vi "TDMS.GetIteration.vi"(8 "error in (no error)":errorcluster, 11 "Data":path) -> (0 "error out":errorcluster, 2 "Iteration":i32)   [LabVIEW 2014, in "NIAnalysis.lvlib"]
uses:
  NIAnalysis.lvlib
  Constants.vi
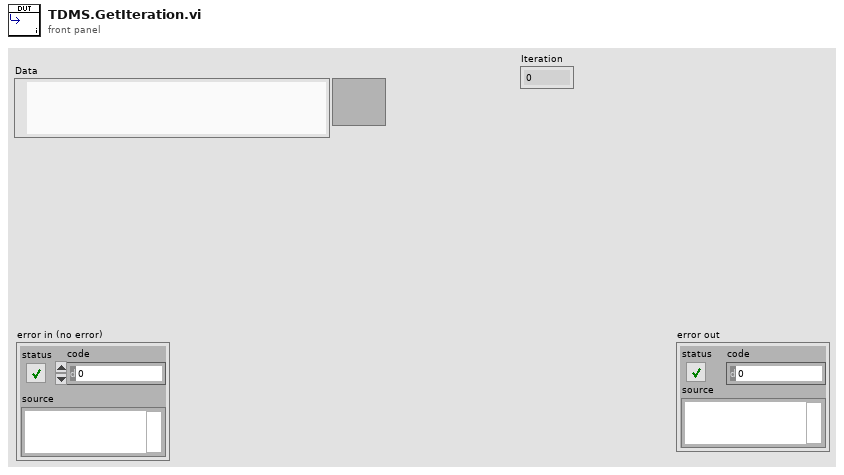
[diagram p1: front panel]
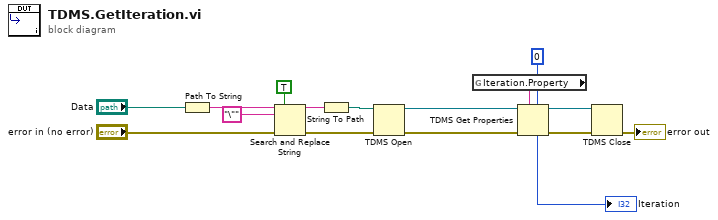
[diagram p0: block diagram]
diagram:
  n1 = Path To String(path="Data") -> (string=w15:string)
  n2 = Search and Replace String(replace all?=TRUE ("replace all? (F)"), input string=w15, search string="\"", error in="error in (no error)") -> (result string=w16:string, error out=w10:errorcluster)  [unwired: 4 in, 2 out]
  n3 = String To Path(string=w16) -> (path=w11:path)
  n4 = TDMS Open(8:w10, 11:w11) -> (0:w6:errorcluster, 3:w7:refnum<k34>)  [unwired: 5 in]
  n5 = global read "Constants.vi" "Iteration.Property"() -> (w8:string)
  n6 = TDMS Get Properties(5:0 ("Iteration"), 7:w8, 8:w6, 11:w7) -> (0:w3:errorcluster, 3:w2:refnum<k34>, 4:→"Iteration":i32)  [unwired: 2 in, 3 out]
  n7 = TDMS Close(8:w3, 11:w2) -> (0:→"error out":errorcluster)  [unwired: 1 out]
